vi "F Dwf Analog Out Node Play Data.vi"(6 "cdData":i32, 7 "rgdData":dbl, 8 "error in (no error)":errorcluster, 9 "node":i32, 10 "idxChannel":i32, 11 "hdwf":i32) -> (0 "error out":errorcluster, 3 "function return":i32, 5 "rgdData out":dbl)   [LabVIEW 2019, in "Olasdwf.lvlib"]
doc: "DWFAPI int FDwfAnalogOutNodePlayData(HDWF hdwf, int idxChannel, AnalogOutNode node, double *rgdData, int cdData);"
uses:
  Olasdwf.lvlib
  Windows/System32/dwf.dll
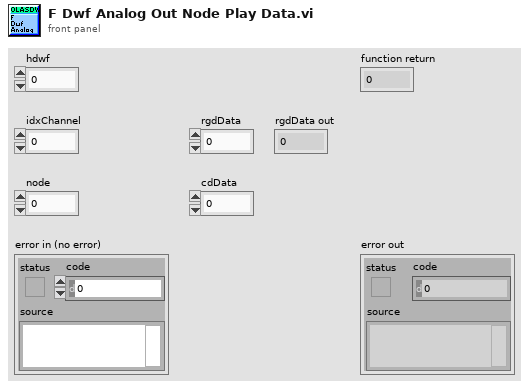
[diagram p1: front panel]
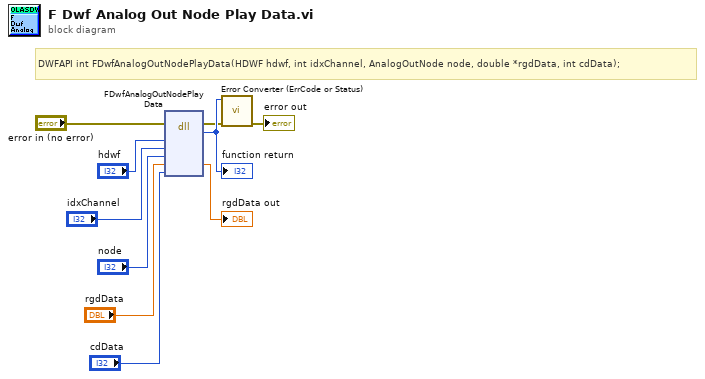
[diagram p0: block diagram]
diagram:
  # "DWFAPI int FDwfAnalogOutNodePlayData(HDWF hdwf, int idxChannel, AnalogOutNode node, double *rgdData, int cdData);"
  n1 = dll-call lib="C:/Windows/System32/dwf.*" fn="FDwfAnalogOutNodePlayData"(error in="error in (no error)", "hdwf"="hdwf", "idxChannel"="idxChannel", "node"="node", "rgdData"="rgdData", "cdData"="cdData") -> (error out=w2:errorcluster, w10:i32, "rgdData"=→"rgdData out":dbl)  [unwired: 6 in, 1 out]
  "function return" <- w10
  n2 = call "Error Converter (ErrCode or Status).vi"("error in (no error)"=w2, "error code"=w10) -> ("error out"=→"error out":errorcluster)  [unwired: 9 in]
